vi "LIA Fgen Arbitrary Waveform (Dual Channel).vi"() -> ()   [LabVIEW 2017]
doc: "This example shows how to use the Arbitrary Waveform mode to generate on two channels."
uses:
  <instrlib>/niFgen/niFgen.llb/niFgen Output Mode.ctl
  <instrlib>/niFgen/niFgen.llb/niFgen Waveform Type.ctl
panel:
  in  "Frequency":dbl=100000.0 format="%_6p"
  in  "Amplitude":dbl=1.0 format="%_4g"
  in  "Stop":bool
  in  "FGEN Resource Name":refnum<k15>="Dev4"
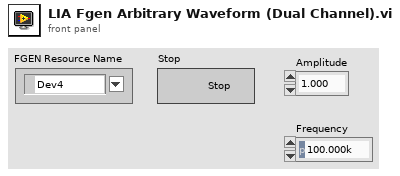
[diagram p1: front panel]
types:
  T1 = typedef "niFgen Waveform Type.ctl" = i32
  T2 = typedef "niFgen Output Mode.ctl" = u32
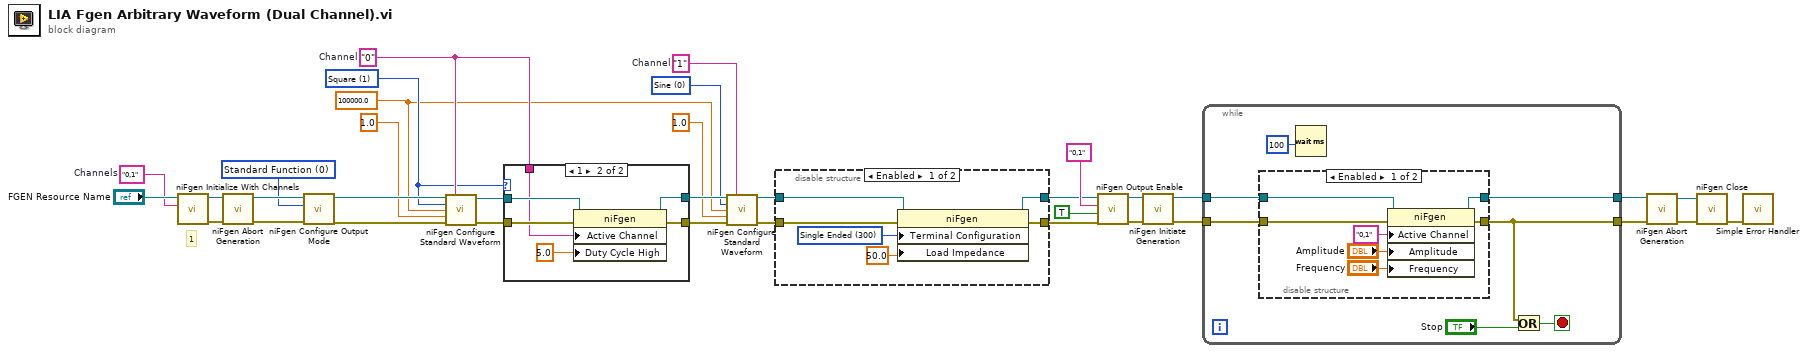
[diagram p0: block diagram]
diagram:
  w12 = "1"  # Channel
  w14 = T1 0 items=["Sine", "Square", "Triangle", "Ramp Up", "Ramp Down", "DC", "Noise", "User"] ("Waveform")
  w1 = 100000.0 ("Frequency")
  w2 = T1 1 items=["Sine", "Square", "Triangle", "Ramp Up", "Ramp Down", "DC", "Noise", "User"] ("Waveform")
  w19 = "0"  # Channel
  w26 = T2 0 items=["Standard Function", "Frequency List", "Arbitrary Waveform", "Arbitrary Sequence", "Script"] ("Output Mode")
  w31 = "0,1"  # Channels
  # "1"
  n1 = call <instrlib>:"niFgen Initialize With Channels.vi"("Channel Name"=w31, "Resource Name"="FGEN Resource Name") -> ("error out"=w30:errorcluster, "Instrument Handle Out"=w29:refnum<k15>)  [unwired: 8 in]
  n2 = call <instrlib>:"niFgen Abort Generation.vi"("error in (no error)"=w30, "Instrument Handle"=w29) -> ("error out"=w28:errorcluster, "Instrument Handle Out"=w27:refnum<k15>)  [unwired: 8 in]
  n3 = call <instrlib>:"niFgen Configure Output Mode.vi"("error in (no error)"=w28, "Output Mode (default: 0=Standard Function)"=w26, "Instrument Handle"=w27) -> ("error out"=w21:errorcluster, "Instrument Handle Out"=w22:refnum<k15>)  [unwired: 6 in]
  n4 = call <instrlib>:"niFgen Configure Standard Waveform.vi"("Instrument Handle"=w22, "Channel Name"=w19, "Waveform"=w2, "Frequency"=w1, "Amplitude"=1.0, "error in (no error)"=w21) -> ("Instrument Handle Out"=w24:refnum<k15>, "error out"=w23:errorcluster)  [unwired: 8 in]
  n5 = case shown="1" w2 {
    tunnel: w24 -> [w37 w43]
    tunnel: w23 -> [w36 w42]
    tunnel: w19 -> [_ w41]
    tunnel: [w37 w39] -> w15
    tunnel: [w36 w38] -> w11
    frame Default {
    }
    frame 1 {
      n6 = property class="niFgen"(reference=w43, error in=w42, "Active Channel"=w41, "Duty Cycle High"=5.0 ("Standard Function:Duty Cycle High")) -> (reference out=w39:refnum<k15>, error out=w38:errorcluster)
    }
  }
  n7 = call <instrlib>:"niFgen Configure Standard Waveform.vi"("Instrument Handle"=w15, "Channel Name"=w12, "Waveform"=w14, "Frequency"=w1, "Amplitude"=1.0, "error in (no error)"=w11) -> ("Instrument Handle Out"=w4:refnum<k15>, "error out"=w10:errorcluster)  [unwired: 8 in]
  n8 = disable-structure shown="Enabled" {
    disable-tunnel: w10 -> [w49 w50]
    disable-tunnel: [w48 w50] -> w5
    disable-tunnel: w4 -> [w47 w51]
    disable-tunnel: [w46 w51] -> w3
    frame Enabled {
      w45 = 300 items=["Single Ended"=300, "Differential"=301] ("Output:Terminal Configuration")
      n9 = property class="niFgen"(reference=w47, error in=w49, "Terminal Configuration"=w45, "Load Impedance"=50.0 ("Output:Load Impedance")) -> (reference out=w46:refnum<k15>, error out=w48:errorcluster)
    }
    frame Disabled {
    }
  }
  n10 = call <instrlib>:"niFgen Output Enable.vi"("error in (no error)"=w5, "Output Enable (default: True)"=TRUE ("output enable"), "Channel Name"="0,1", "Instrument Handle"=w3) -> ("error out"=w16:errorcluster, "Instrument Handle Out"=w17:refnum<k15>)  [unwired: 6 in]
  n11 = call <instrlib>:"niFgen Initiate Generation.vi"("error in (no error)"=w16, "Instrument Handle"=w17) -> ("error out"=w8:errorcluster, "Instrument Handle Out"=w6:refnum<k15>)  [unwired: 8 in]
  n12 = while {
    tunnel: [w54] -> w9
    tunnel: w8 -> [w55]
    tunnel: [w52] -> w7
    tunnel: w6 -> [w53]
    stop <- w56 stop-if-true
    n13 = disable-structure shown="Enabled" {
      disable-tunnel: w55 -> [w65 w66]
      disable-tunnel: [w64 w66] -> w54
      disable-tunnel: w53 -> [w63 w67]
      disable-tunnel: [w62 w67] -> w52
      frame Enabled {
        n14 = property class="niFgen"(reference=w63, error in=w65, "Active Channel"="0,1", "Amplitude"="Amplitude", "Frequency"="Frequency") -> (reference out=w62:refnum<k15>, error out=w64:errorcluster)
      }
      frame Disabled {
      }
    }
    n15 = Wait (ms)(milliseconds to wait=u32 100 ("millisecond multiple")) -> ()  [unwired: 1 out]
    n16 = Or(x=w54, y="Stop") -> (x .or. y?=w56:bool)
  }
  n17 = call <instrlib>:"niFgen Abort Generation.vi"("error in (no error)"=w9, "Instrument Handle"=w7) -> ("error out"=w35:errorcluster, "Instrument Handle Out"=w34:refnum<k15>)  [unwired: 8 in]
  n18 = call <instrlib>:"niFgen Close.vi"("error in (no error)"=w35, "Instrument Handle"=w34) -> ("error out"=w33:errorcluster)  [unwired: 9 in]
  n19 = call <vilib>:"Simple Error Handler.vi"("error in (no error)"=w33) -> ()  [unwired: 4 in, 5 out]
